vi "test2-SyncMessageWithError.vi"(8 "error in (no error)":errorcluster, 11 "TestCase in":refnum<class "testcase-CSMMessage.lvclass">) -> (0 "error out":errorcluster, 3 "TestCase out":refnum<class "testcase-CSMMessage.lvclass">)   [LabVIEW 2017, in "testcase-CSMMessage.lvclass"]
uses:
  testcase-CSMMessage.lvclass
  src/user.lib/_NEVSTOP/Communicable State Machine(CSM)/AdvanceAPI/CSM - Make String Arguments Safe.vi
  src/user.lib/_NEVSTOP/Communicable State Machine(CSM)/AdvanceAPI/CSM - Keywords.vi
  <vilib>/addons/_JKI Toolkits/VI Tester/TestCase.llb/TestCase.lvclass
  src/user.lib/_NEVSTOP/Communicable State Machine(CSM)/Communicable State Machine.lvlib
  C:/Program Files (x86)/National Instruments/LabVIEW 2017/vi.lib/addons/_JKI Toolkits/VI Tester/TestCase.llb/TestCase.lvclass
panel:
  out "Loopcount":i32
  out "Source CSM modules":string[](array[string])
  out "concatenated string":string
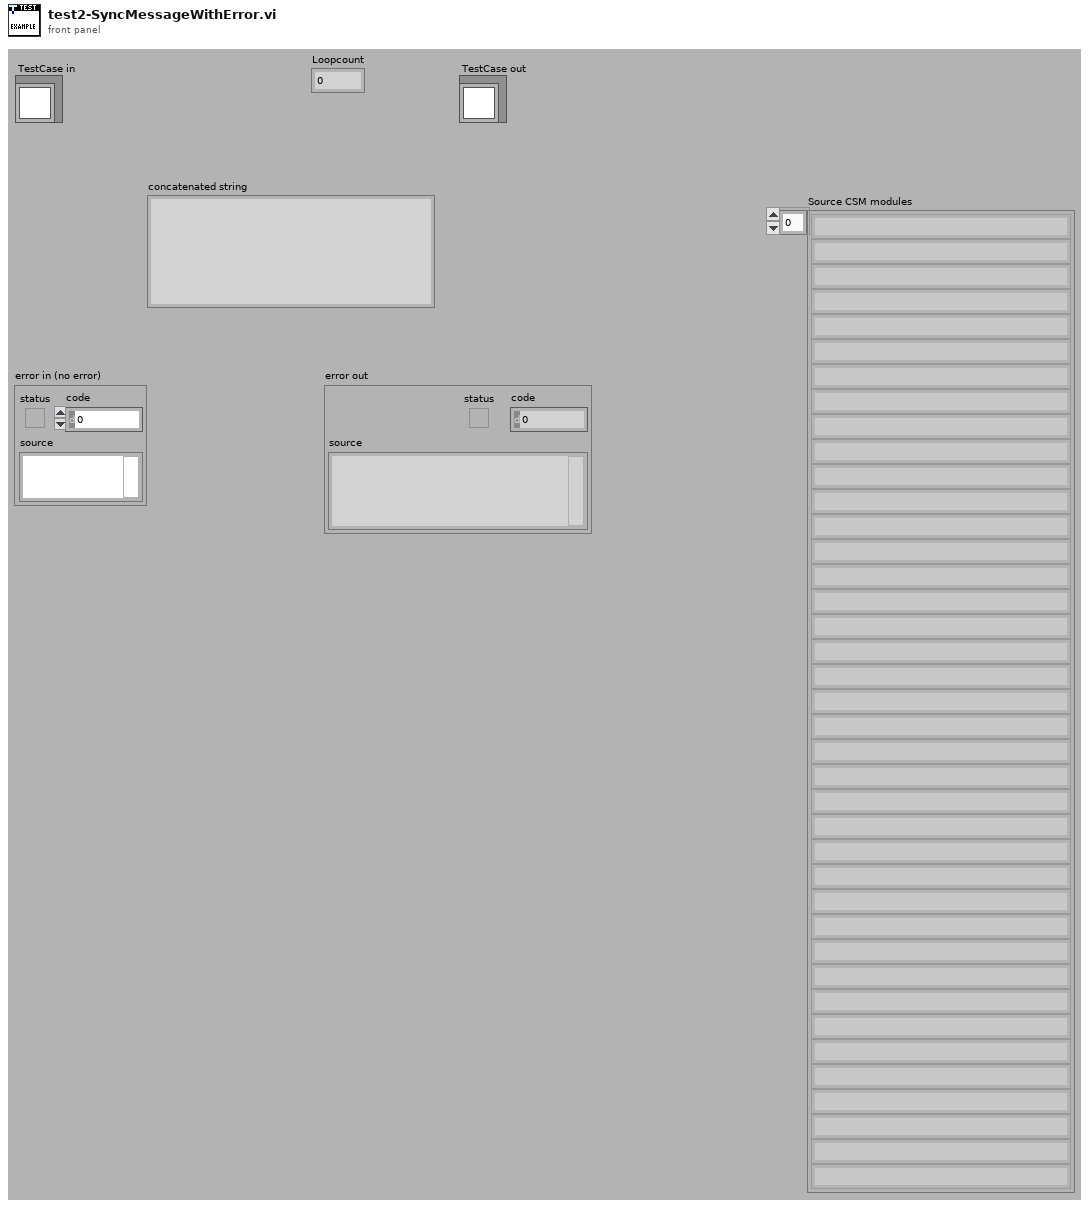
[diagram p1: front panel]
types:
  T1 = cluster{"Arguments":string, "Response":string, "error":errorcluster}
  T2 = cluster{"status":bool, "code":bool, "source":bool}
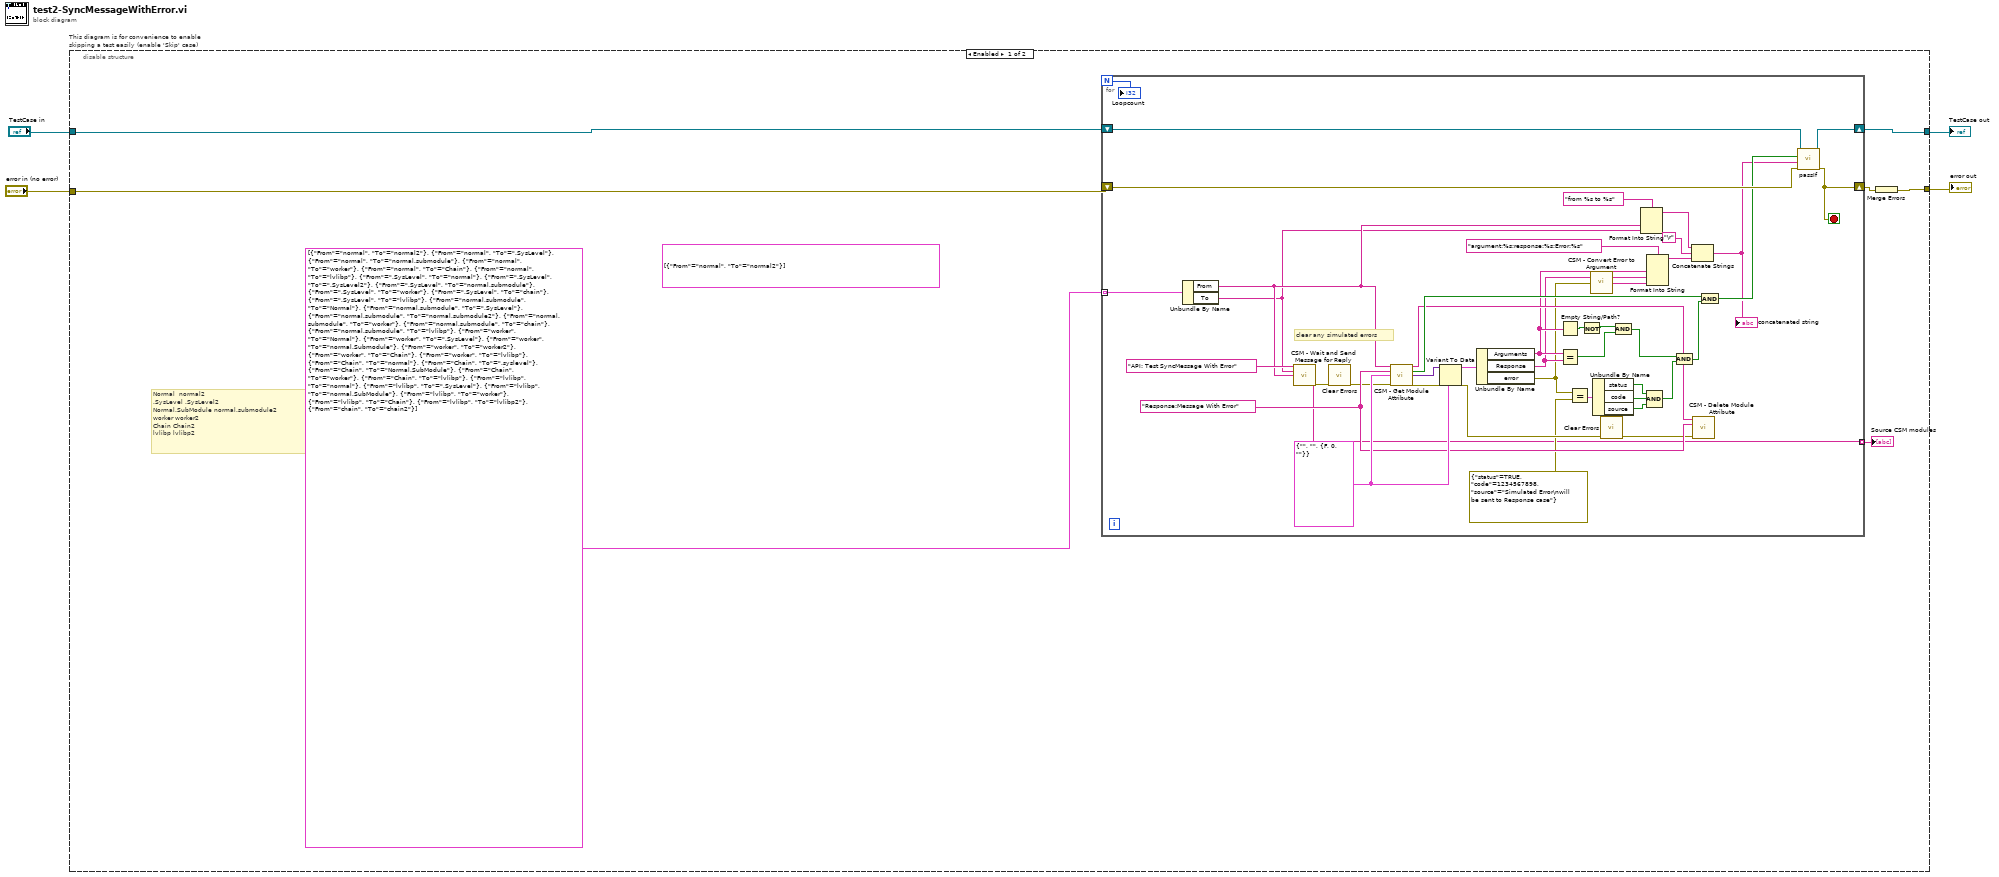
[diagram p0: block diagram]
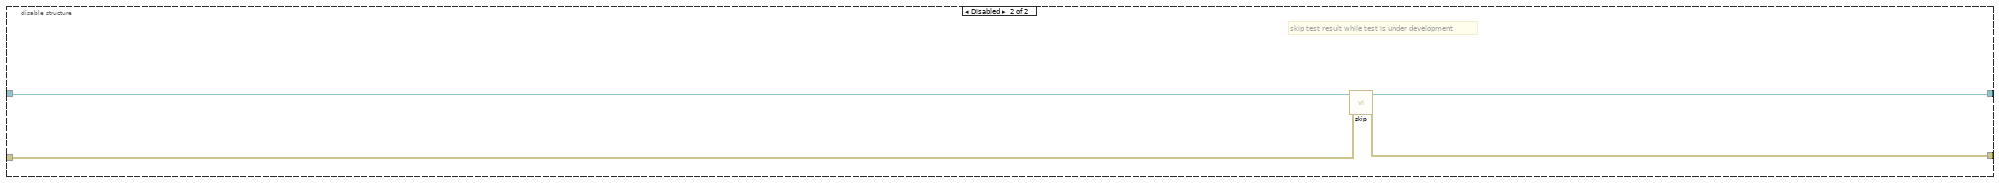
[diagram p2: hidden frame]
diagram:
  n1 = disable-structure "This diagram is for convenience to enable skipping a test easily (enable 'Skip' case)" shown="Enabled" {
    disable-tunnel: "TestCase in" -> [w11 w58]
    disable-tunnel: [w10 w56] -> w1
    disable-tunnel: [w7 w57] -> w3
    disable-tunnel: "error in (no error)" -> [w8 w55]
    frame Enabled {
      (unwired) cluster{"From":string, "To":string}[] [{"From"="normal", "To"="normal2"}]
      # "Normal  normal2\n.SysLevel .SysLevel2\nNormal.SubModule normal.submodule2\nworker worker2\nChain Chain2\nlvlibp lvlibp2"
      n2 = for {
        N -> [w12]
        tunnel: cluster{"From":string, "To":string}[] [{"From"="normal", "To"="normal2"}, {"From"="normal", "To"=".SysLevel"}, {"From"="normal", "To"="normal.submodule"}, {"From"="normal", "To"="worker"}, {"From"="normal", "To"="Chain"}, {"From"="normal", "To"="lvlibp"}, {"From"=".SysLevel", "To"="normal"}, {"From"=".SysLevel", "To"=".SysLevel2"}, {"From"=".SysLevel", "To"="normal.submodule"}, {"From"=".SysLevel", "To"="worker"}, {"From"=".SysLevel", "To"="chain"}, {"From"=".SysLevel", "To"="lvlibp"}, {"From"="normal.submodule", "To"="Normal"}, {"From"="normal.submodule", "To"=".SysLevel"}, {"From"="normal.submodule", "To"="normal.submodule2"}, {"From"="normal.submodule", "To"="worker"}, {"From"="normal.submodule", "To"="chain"}, {"From"="normal.submodule", "To"="lvlibp"}, {"From"="worker", "To"="Normal"}, {"From"="worker", "To"=".SysLevel"}, {"From"="worker", "To"="normal.Submodule"}, {"From"="worker", "To"="worker2"}, {"From"="worker", "To"="Chain"}, {"From"="worker", "To"="lvlibp"}, {"From"="Chain", "To"="normal"}, {"From"="Chain", "To"=".syslevel"}, {"From"="Chain", "To"="Normal.SubModule"}, {"From"="Chain", "To"="worker"}, {"From"="Chain", "To"="lvlibp"}, {"From"="lvlibp", "To"="normal"}, {"From"="lvlibp", "To"=".SysLevel"}, {"From"="lvlibp", "To"="normal.SubModule"}, {"From"="lvlibp", "To"="worker"}, {"From"="lvlibp", "To"="Chain"}, {"From"="lvlibp", "To"="lvlibp2"}, {"From"="chain", "To"="chain2"}] -> [w43] mode=indexing
        shift-right: [w53] -> w10
        shift-left: w11 -> [w54]
        shift-right: [w25] -> w9
        shift-left: w8 -> [w52]
        tunnel: [w13] -> w5 mode=indexing
        stop <- w25 stop-if-true
        w49 = T1 {"Arguments"="", "Response"="", "error"={"status"=FALSE, "code"=0, "source"=""}}
        w40 = "Response:Message With Error" ("State")
        # "clear any simulated errors"
        n3 = Unbundle By Name(w43) -> ("From"=w15:string, "To"=w14:string)
        n4 = call "CSM - Wait and Send Message for Reply.vi"("State"="API: Test SyncMessage With Error", "Arguments (\"\")"=w14, "Target Module"=w15) -> (">> Source CSM >>"=w13:string, "error out"=w17:errorcluster)  [unwired: 10 in, 1 out]
        n5 = call <vilib>:"Clear Errors.vi"("error in (no error)"=w17) -> ("error out"=w16:errorcluster)  [unwired: 5 in, 1 out]
        n6 = call "CSM - Get Module Attribute.vi"("CSM Name"=w15, "Attribute"=w40, "Default Value (Empty Variant)"=w49, "Error In"=w16) -> ("CSM Name (Dup)"=w41:string, "Found"=w46:bool, "Value"=w48:variant, "error out"=w50:errorcluster)  [unwired: 7 in, 1 out]
        n7 = Variant To Data(error in=w50, type=w49, Variant=w48) -> (data=w47:T1, error out=w27:errorcluster)
        n8 = Unbundle By Name(w47) -> ("Arguments"=w35:string, "Response"=w34:string, "error"=w24:errorcluster)
        n9 = Empty String/Path?(string/path=w35) -> (empty?=w39:bool)
        n10 = Equal?(x=w35, y=w34) -> (x = y?=w37:bool)
        n11 = Equal?(x=w24, y=errorcluster {"status"=TRUE, "code"=1234567898, "source"="Simulated Error\nwill be sent to Response case"} ("error out")) -> (x = y?=w22:T2)
        n12 = Not(x=w39) -> (.not. x?=w38:bool)
        n13 = call "CSM - Convert Error to Argument.vi"("Error"=w24) -> ("Argument"=w33:string)  [unwired: 4 in]
        n14 = Unbundle By Name(w22) -> ("status"=w21:bool, "code"=w20:bool, "source"=w19:bool)
        n15 = call <vilib>:"Clear Errors.vi"("error in (no error)"=w27) -> ("error out"=w26:errorcluster)  [unwired: 5 in, 1 out]
        n16 = And(x=w38, y=w37) -> (x .and. y?=w36:bool)
        n17 = Format Into String(format string="from %s to %s", w15, w14) -> (resulting string=w29:string)  [unwired: 2 in, 1 out]
        n18 = Format Into String(format string="argument:%s;response:%s;Error:%s", w35, w34, w33) -> (resulting string=w32:string)  [unwired: 2 in, 1 out]
        n19 = Compound Arithmetic op=AND(w21, w20, w19) -> (w18:bool)
        n20 = And(x=w36, y=w18) -> (x .and. y?=w45:bool)
        n21 = Concatenate Strings(w29, "\r", w32) -> (w30:string)
        "concatenated string" <- w30
        n22 = call "CSM - Delete Module Attribute.vi"("CSM Name"=w41, "Attribute"=w40, "Error In"=w26) -> ()  [unwired: 9 in, 4 out]
        n23 = And(x=w46, y=w45) -> (x .and. y?=w44:bool)
        n24 = call-dynamic "passIf.vi"("error in (no error)"=w52, "message (\"\")"=w30, "pass"=w44, "TestCase in"=w54) -> ("error out"=w25:errorcluster, "TestCase out"=w53:refnum<class "testcase-CSMMessage.lvclass">)  [unwired: 6 in]
        "Loopcount" <- w12
      }
      "Source CSM modules" <- w5
      n25 = Merge Errors(w9) -> (w7:errorcluster)
    }
    frame Disabled {
      # "skip test result while test is under development"
      n26 = call <vilib>:"skip.vi"("error in (no error)"=w55, "TestCase in"=w58) -> ("error out"=w57:errorcluster, "TestCase out"=w56:refnum<class "testcase-CSMMessage.lvclass">)  [unwired: 8 in]
    }
  }
  "error out" <- w3
  "TestCase out" <- w1
